vi "SVFA Power Spectrum.vi"   [LabVIEW 2017]
doc: "Computes the power spectrum of <B>scaled signal [EU]</B>. Use the power spectrum to quantify signal components as a function of frequency. Wire data to the <B>scaled signal [EU]</B> input to determine the polymorphic instance to use or manually select the instance."
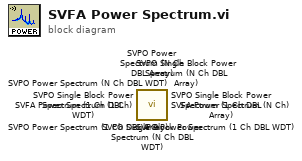
[diagram p0: block diagram]
diagram:
  n1 = call <vilib>:"SVPO Single Block Power Spectrum (N Ch DBL WDT).vi"() -> ()  [unwired: 18 in, 2 out]
  n2 = call <vilib>:"SVPO Single Block Power Spectrum (N Ch DBL Array).vi"() -> ()  [unwired: 18 in, 2 out]
  n3 = call <vilib>:"SVPO Single Block Power Spectrum (1 Ch DBL WDT).vi"() -> ()  [unwired: 18 in, 2 out]
  n4 = call <vilib>:"SVPO Single Block Power Spectrum (1 Ch DBL Array).vi"() -> ()  [unwired: 18 in, 2 out]
  n5 = call <vilib>:"SVPO Power Spectrum (N Ch DBL WDT).vi"() -> ()  [unwired: 17 in, 3 out]
  n6 = call <vilib>:"SVPO Power Spectrum (1 Ch DBL WDT).vi"() -> ()  [unwired: 17 in, 3 out]
  n7 = call <vilib>:"SVPO Power Spectrum (N Ch DBL Array).vi"() -> ()  [unwired: 17 in, 3 out]
  n8 = call <vilib>:"SVPO Power Spectrum (1 Ch DBL Array).vi"() -> ()  [unwired: 17 in, 3 out]
  n9 = call <vilib>:"SVFA Power Spectrum (1 Ch).vi"() -> ()  [unwired: 14 in, 6 out]
  n10 = call <vilib>:"SVFA Power Spectrum (N Ch).vi"() -> ()  [unwired: 14 in, 6 out]
